vi "Configure Fixture Simulator.vi"(0 "VISA resource name":refnum<visa-resource-name>, 1 "Channel (1)":i32=1, 2 "Balance Device Type (0: Unbalance - Balance)":u16(ring) items=["Unbalance - Balance", "Balance - Balance", "Unbalance - Unbalance - Balance", "Balance"], 3 "Display Property (F: Disable)":bool, 5 "Fixture Simulator State (F: Disable)":bool, 7 "Port 1 (1)":i32=1, 9 "Port 2 (2)":i32=2, 11 "error in (no error)":errorcluster, 12 "Port 3 (3)":i32=3, 13 "Port 4 (4)":i32=4) -> (4 "VISA resource name out":refnum<visa-resource-name>, 15 "error out":errorcluster)   [LabVIEW 2018, in "Agilent ENA Series.lvlib"]
doc: "Configures the fixture simulator.\n\nNote:\nThe control Display Property does not support model E5080A."
uses:
  Agilent ENA Series.lvlib
panel:
  # "Note:\nThe control Display Property does not support model E5080A."
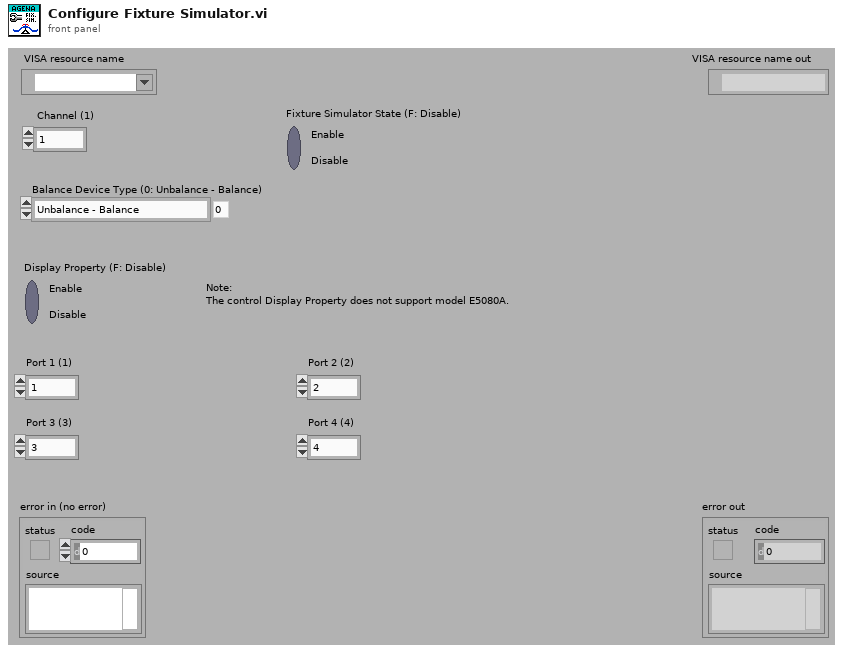
[diagram p1: front panel]
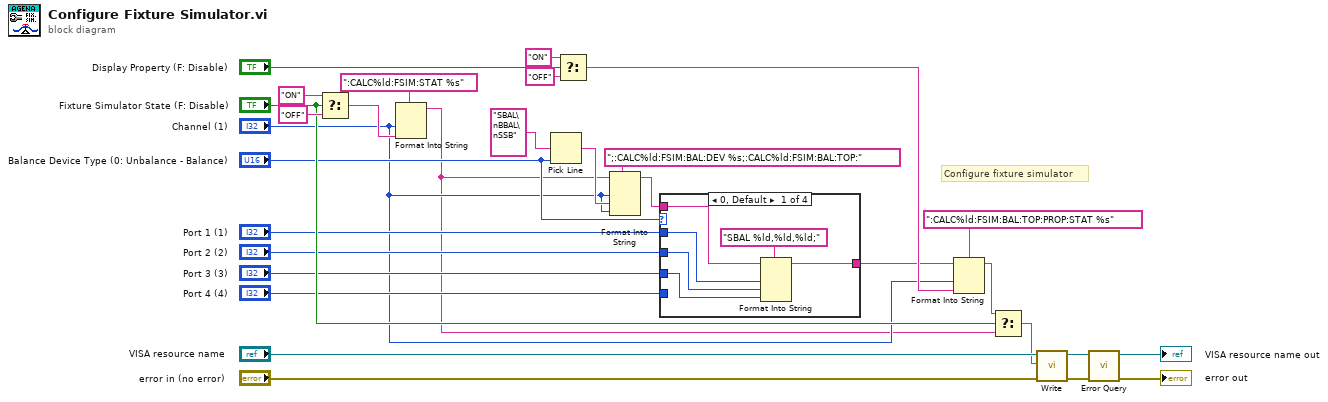
[diagram p0: block diagram]
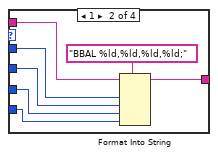
[diagram p2: hidden frame]
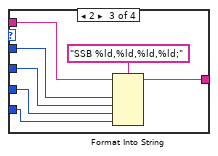
[diagram p3: hidden frame]
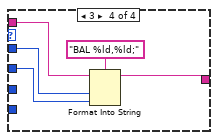
[diagram p4: hidden frame]
diagram:
  # "Configure fixture simulator"
  n1 = Select(t="ON", s="Fixture Simulator State (F: Disable)", f="OFF") -> (s? t:f=w26:string)
  n2 = Format Into String(format string=":CALC%ld:FSIM:STAT %s", "Channel (1)", w26) -> (resulting string=w5:string)  [unwired: 2 in, 1 out]
  n3 = Pick Line(multi-line string="SBAL\nBBAL\nSSB", line index="Balance Device Type (0: Unbalance - Balance)") -> (output string=w21:string)  [unwired: 1 in]
  n4 = Select(t="ON", s="Display Property (F: Disable)", f="OFF") -> (s? t:f=w9:string)
  n5 = Format Into String(format string=";:CALC%ld:FSIM:BAL:DEV %s;:CALC%ld:FSIM:BAL:TOP:", initial string=w5, "Channel (1)", w21, "Channel (1)") -> (resulting string=w19:string)  [unwired: 1 in, 1 out]
  n6 = case shown="0, Default" "Balance Device Type (0: Unbalance - Balance)" {
    tunnel: w19 -> [w35 w42 w49 w53]
    tunnel: "Port 1 (1)" -> [w34 w41 w48 w52]
    tunnel: "Port 2 (2)" -> [w33 w40 w47 w51]
    tunnel: "Port 3 (3)" -> [w32 w39 w46 _]
    tunnel: "Port 4 (4)" -> [_ w37 w44 _]
    tunnel: [w31 w38 w45 w54] -> w8
    frame 0, Default {
      n7 = Format Into String(format string="SBAL %ld,%ld,%ld;", initial string=w35, w34, w33, w32) -> (resulting string=w31:string)  [unwired: 1 in, 1 out]
    }
    frame 1 {
      n8 = Format Into String(format string="BBAL %ld,%ld,%ld,%ld;", initial string=w42, w41, w40, w39, w37) -> (resulting string=w38:string)  [unwired: 1 in, 1 out]
    }
    frame 2 {
      n9 = Format Into String(format string="SSB %ld,%ld,%ld,%ld;", initial string=w49, w48, w47, w46, w44) -> (resulting string=w45:string)  [unwired: 1 in, 1 out]
    }
    frame 3 {
      n10 = Format Into String(format string="BAL %ld,%ld;", initial string=w53, w52, w51) -> (resulting string=w54:string)  [unwired: 1 in, 1 out]
    }
  }
  n11 = Format Into String(format string=":CALC%ld:FSIM:BAL:TOP:PROP:STAT %s", initial string=w8, "Channel (1)", w9) -> (resulting string=w7:string)  [unwired: 1 in, 1 out]
  n12 = Select(t=w7, s="Fixture Simulator State (F: Disable)", f=w5) -> (s? t:f=w14:string)
  n13 = call "Write.vi"("error in (no error)"="error in (no error)", "String ()"=w14, "VISA resource name"="VISA resource name") -> ("error out"=w3:errorcluster, "VISA resource name out"=w4:refnum<visa-resource-name>)  [unwired: 6 in, 1 out]
  n14 = call "Error Query.vi"("error in (no error)"=w3, "VISA resource name"=w4) -> ("error out"=→"error out":errorcluster, "VISA resource name out"=→"VISA resource name out":refnum<visa-resource-name>)  [unwired: 6 in, 2 out]
